vi "Generate Signal.vi"(8 "error in (no error)":errorcluster, 9 "?":dbl=1.0, 10 "Frequency (1000 Hz)":dbl=1000.0, 11 "Function Generator in":refnum<class "Function Generator.lvclass">) -> (0 "error out":errorcluster, 3 "Function Generator out":refnum<class "Function Generator.lvclass">)   [LabVIEW 2015, in "Hardware.lvlib" / "Function Generator.lvclass"]
uses:
  Function Generator.lvclass
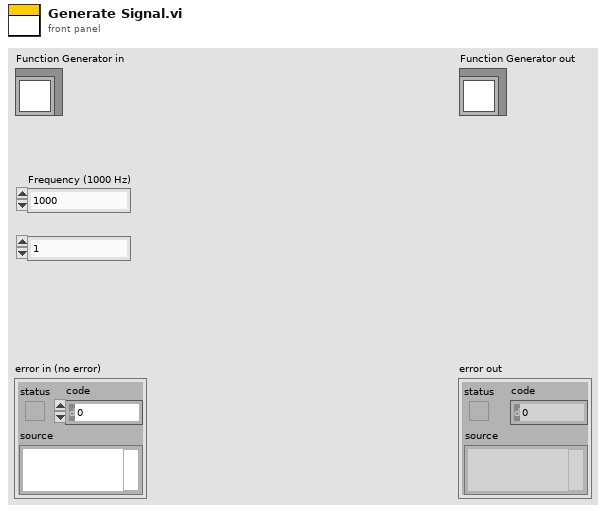
[diagram p1: front panel]
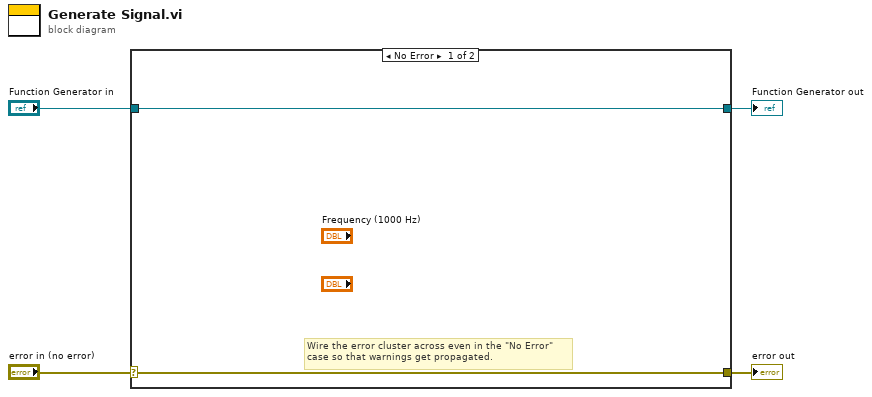
[diagram p0: block diagram]
diagram:
  n1 = case shown="No Error" "error in (no error)" {
    selector: "error in (no error)" -> [w5 w8]
    tunnel: [w5 w8] -> w3
    tunnel: [w6 w7] -> w1
    tunnel: "Function Generator in" -> [w6 w7]
    frame No Error {
      # "Wire the error cluster across even in the \"No Error\"\ncase so that warnings get propagated."
    }
    frame Error {
    }
  }
  "error out" <- w3
  "Function Generator out" <- w1
